vi "1000m_sub_frame.vi"(7 "Case select":string, 8 "felharmonikus N":i32=2, 9 "SNR window width [Hz]":dbl=0.4 format="%#_13g", 11 "path to binary file":path) -> (3 "output cluster":T1)   [LabVIEW 2017]
uses:
  <vilib>/Utility/file.llb/Read Delimited Spreadsheet (string).vi
  <vilib>/regexp/Match Regular Expression.xnode
panel:
  out "impulse szum/mean":cluster{"X":dbl, "Y":dbl}[](graph)
  out "Array":T2(array[cluster])
  out "header":T3
  out "impulse szum/time (bigger better)":cluster{"X":dbl, "Y":dbl}[](graph)
  out "X SNR 2":cluster{"X":dbl, "Y":dbl}[](graph)
  out "resultant SNR":cluster{"X":dbl, "Y":dbl}[](graph)
  out "X SNR":cluster{"X":dbl, "Y":dbl}[](graph)
  out "impulse mean":cluster{"X":dbl, "Y":dbl}[](graph)
  out "impulse sd":cluster{"X":dbl, "Y":dbl}[](graph)
  out "impulse szum":cluster{"X":dbl, "Y":dbl}[](graph)
  out "enable":bool
  out "end":timestamp
  out "start":timestamp
  out "state":string
  out "saved":string
  out "all rows":string[][](array[string])
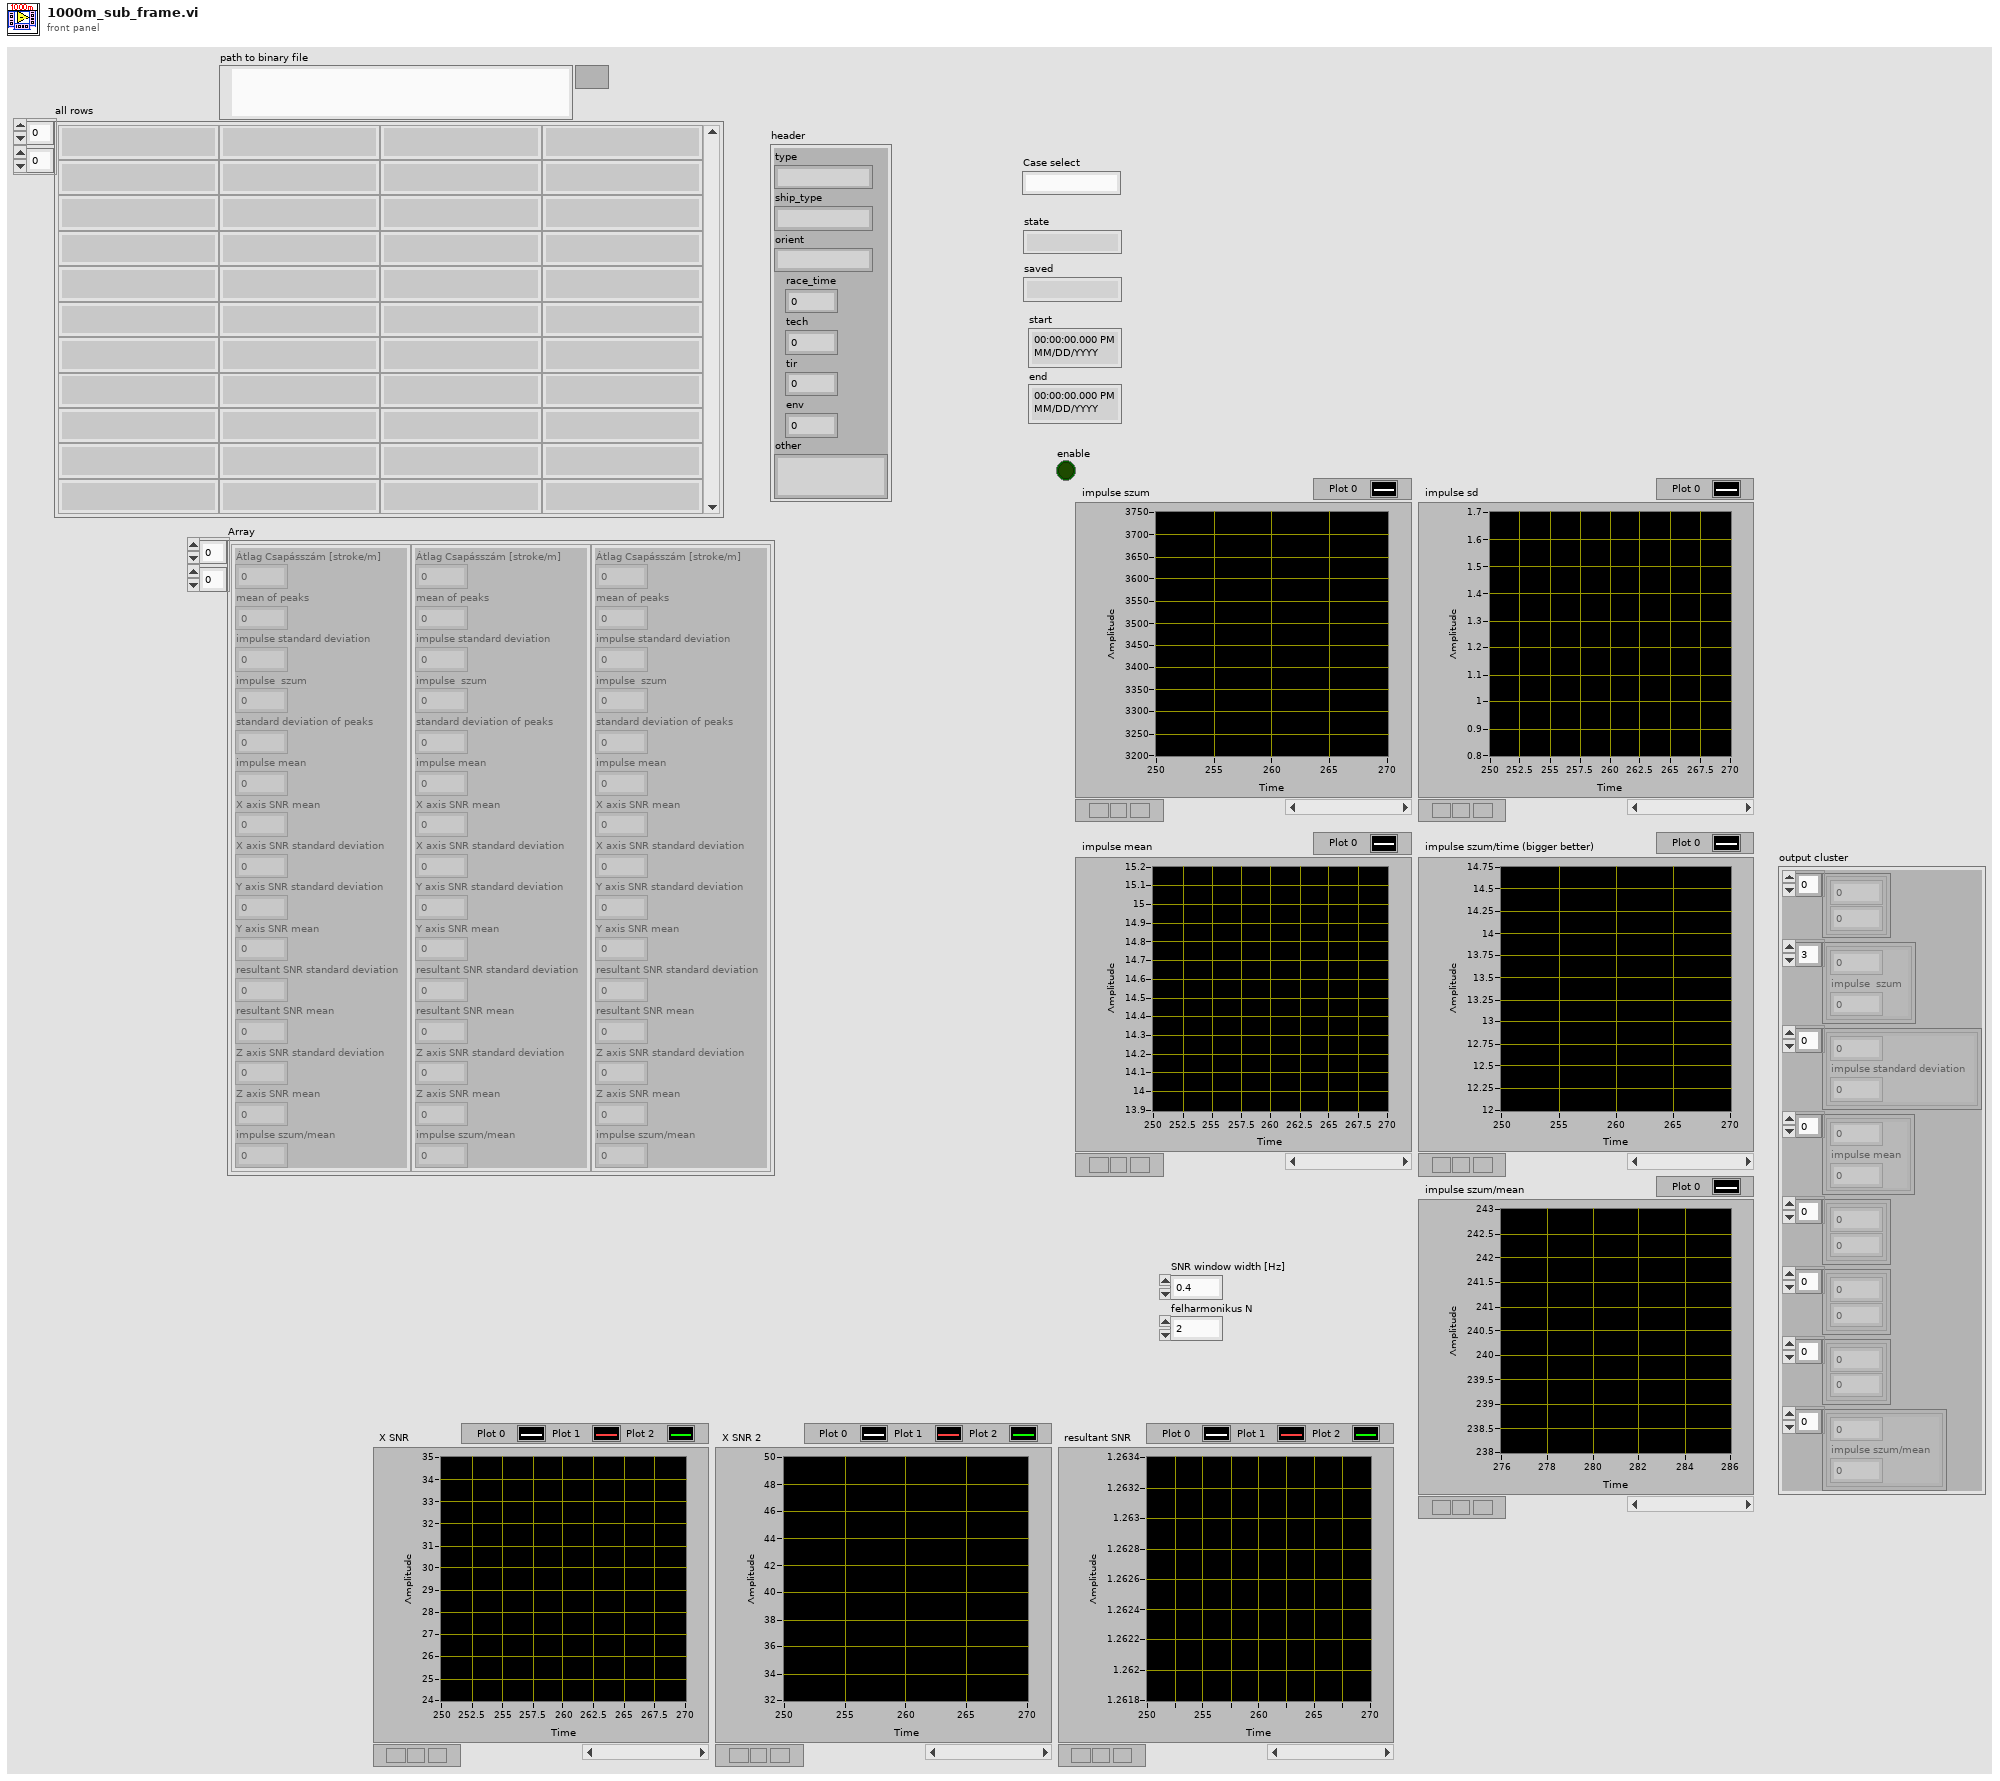
[diagram p1: front panel]
types:
  T1 = cluster{cluster{dbl, dbl}[], cluster{dbl, "impulse  szum":dbl}[], cluster{dbl, "impulse standard deviation":dbl}[], cluster{dbl, "impulse mean":dbl}[], cluster{dbl, dbl}[], cluster{dbl, dbl}[], cluster{dbl, dbl}[], cluster{dbl, "impulse szum/mean":dbl}[]}
  T2 = cluster{"Átlag Csapásszám [stroke/m]":dbl, "mean of peaks":dbl, "impulse standard deviation":dbl, "impulse  szum":dbl, "standard deviation of peaks":dbl, "impulse mean":dbl, "X axis SNR mean":dbl, "X axis SNR standard deviation":dbl, "Y axis SNR standard deviation":dbl, "Y axis SNR mean":dbl, "resultant SNR standard deviation":dbl, "resultant SNR mean":dbl, "Z axis SNR standard deviation":dbl, "Z axis SNR mean":dbl, "impulse szum/mean":dbl}[][]
  T3 = cluster{"type":string, "ship_type":string, "orient":string, "race_time":dbl, "tech":dbl, "tir":dbl, "env":dbl, "other":string}
  T4 = typedef "control_time_informations.ctl" = cluster{"starting time":timestamp, "ending time":timestamp, "dt[s]":dbl, "sampling rate [Hz]":dbl, "length":dbl}
  T5 = typedef "control_measurement_settings.ctl" = cluster{"sampling frequency [Hz]":dbl, "measurement interval [± g]":i32, "high precision?":bool, "number of pages":i32, "rate code":i32, "range code":i32, "id":i32}
  T6 = cluster{"statistics":cluster{"mean of x axis acceleration":dbl, "standard devation of x axis acceleration":dbl, "mean of y axis acceleration":dbl, "standard devation of y axis acceleration":dbl, "mean of z axis acceleration":dbl, "standard devation of z axis acceleration":dbl, "mean of magnitude of acceleration":dbl, "standard devation of magnitude of acceleration":dbl}, "time informations":T4, "actigraph settings":T5}
  T7 = cluster{"path to binary file":path, "Start Cursor":timestamp, "Sec":dbl, "crossing level":dbl, "threshold":dbl, "avg window size":i32, "peak detect width":i32, "invert":bool, "SNR window width [Hz]":dbl, "felharmonikus N":i32, "End cursor":timestamp}
  T8 = cluster{"Átlag Csapásszám [stroke/m]":dbl, "mean of peaks":dbl, "impulse standard deviation":dbl, "impulse  szum":dbl, "standard deviation of peaks":dbl, "impulse mean":dbl, "X axis SNR mean":dbl, "X axis SNR standard deviation":dbl, "Y axis SNR standard deviation":dbl, "Y axis SNR mean":dbl, "resultant SNR standard deviation":dbl, "resultant SNR mean":dbl, "Z axis SNR standard deviation":dbl, "Z axis SNR mean":dbl, "impulse szum/mean":dbl}
  T9 = cluster{"Átlag Csapásszám [stroke/m]":dbl, "mean of peaks":dbl, "impulse standard deviation":dbl, "impulse  szum":dbl, "standard deviation of peaks":dbl, "impulse mean":dbl, "X axis SNR mean":dbl, "X axis SNR standard deviation":dbl, "Y axis SNR standard deviation":dbl, "Y axis SNR mean":dbl, "resultant SNR standard deviation":dbl, "resultant SNR mean":dbl, "Z axis SNR standard deviation":dbl, "Z axis SNR mean":dbl, "impulse szum/mean":dbl}[]
  T10 = cluster{"Sec":dbl, "impulse standard deviation":dbl}
  T11 = cluster{cluster{"Sec":dbl, dbl}[], cluster{"Sec":dbl, "impulse  szum":dbl}[], cluster{"Sec":dbl, "impulse standard deviation":dbl}[], cluster{"Sec":dbl, "impulse mean":dbl}[], cluster{dbl, "SNR":dbl}[], cluster{dbl, "SNR":dbl}[], cluster{dbl, "SNR":dbl}[], cluster{"Sec":dbl, "impulse szum/mean":dbl}[]}
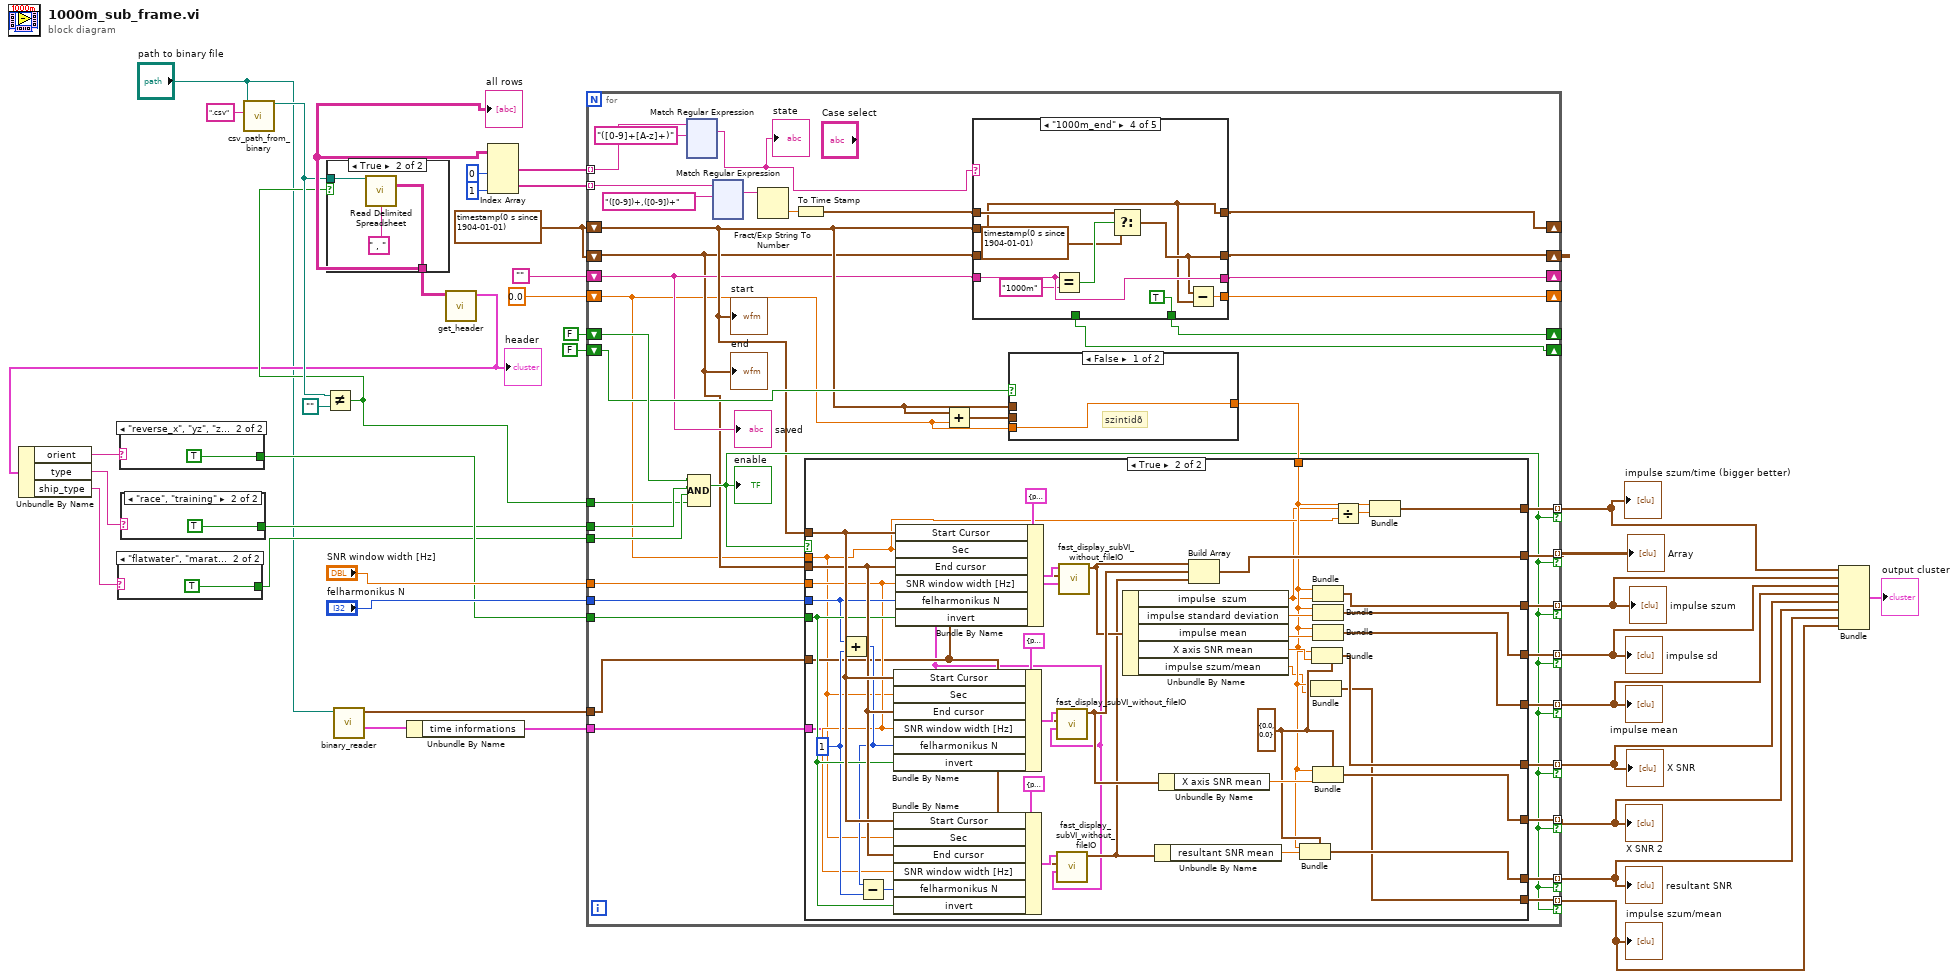
[diagram p0: block diagram]
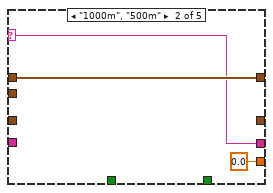
[diagram p3: hidden frame]
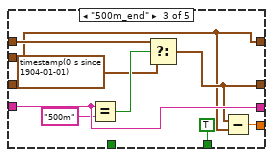
[diagram p4: hidden frame]
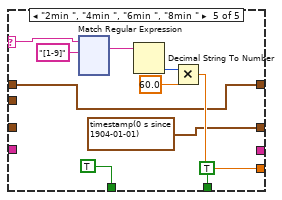
[diagram p5: hidden frame]
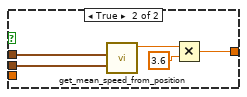
[diagram p6: hidden frame]
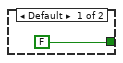
[diagram p9: hidden frame]
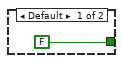
[diagram p10: hidden frame]
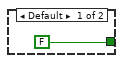
[diagram p11: hidden frame]
diagram:
  w10 = timestamp(0 s since 1904-01-01)
  n1 = call "csv_path_from_binary.vi"("extension"=".csv", "path to binary file"="path to binary file") -> ("path to spec. ext."=w14:path)  [unwired: 9 in]
  n2 = Not Equal?(x=w14, y=path "") -> (x != y?=w13:bool)
  n3 = case shown="True" w13 {
    tunnel: [_ w39] -> w15
    tunnel: w14 -> [_ w38]
    frame False {
    }
    frame True {
      n4 = call-poly <vilib>:"Read Delimited Spreadsheet.vi"("file path (dialog if empty)"=w38, "delimiter (\\t)"=" , " ("delimiter (\\t)")) -> ("all rows"=w39:string[][])  [unwired: 8 in, 5 out]
    }
  }
  "all rows" <- w15
  n5 = call "binary_reader.vi"("path to binary file"="path to binary file") -> ("Misc"=w3:T6, "3 axis acceleration in time"=w4:waveform(dbl)[])  [unwired: 6 in, 2 out]
  n6 = Unbundle By Name(w3) -> ("time informations"=w2:T4)
  n7 = call "get_header.vi"("all rows"=w15) -> ("header"=w11:T3)  [unwired: 10 in]
  "header" <- w11
  n8 = Unbundle By Name(w11) -> ("orient"=w29:string, "type"=w20:string, "ship_type"=w18:string)
  n9 = case shown="\"flatwater\", \"marathon\"" w18 {
    tunnel: [FALSE TRUE] -> w17
    frame Default {
    }
    frame "flatwater", "marathon" {
    }
  }
  n10 = case shown="\"reverse_x\", \"yz\", \"z\"" w29 {
    tunnel: [FALSE TRUE] -> w28
    frame Default {
    }
    frame "reverse_x", "yz", "z" {
    }
  }
  n11 = case shown="\"race\", \"training\"" w20 {
    tunnel: [FALSE TRUE] -> w19
    frame Default {
    }
    frame "race", "training" {
    }
  }
  n12 = Index Array(array=w15, index (col) #1=0 ("disabled index (col)"), index (col) #2=1 ("index (col)")) -> (element #1=w36:string[], element #2=w37:string[])  [unwired: 2 in]
  n13 = for {
    tunnel: w37 -> [w83] mode=indexing
    tunnel: w36 -> [w82] mode=indexing
    shift-right: [w51] -> _
    shift-left: w10 -> [w56]
    shift-right: [w52] -> _
    shift-left: w10 -> [w48]
    shift-right: [w50] -> _
    shift-left: "" -> [w55]
    shift-right: [w49] -> _
    shift-left: 0.0 ("Sec") -> [w47]
    shift-right: [w53] -> _
    shift-left: FALSE -> [w69]
    tunnel: "SNR window width [Hz]" -> [w80]
    tunnel: "felharmonikus N" -> [w79]
    tunnel: w28 -> [w78]
    tunnel: [w77] -> w8 mode=indexing if=w62
    tunnel: [w76] -> w26 mode=indexing if=w62
    tunnel: [w75] -> w25 mode=indexing if=w62
    tunnel: [w74] -> w24 mode=indexing if=w62
    tunnel: [w73] -> w23 mode=indexing if=w62
    tunnel: [w72] -> w22 mode=indexing if=w62
    tunnel: [w71] -> w21 mode=indexing if=w62
    tunnel: [w70] -> w27 mode=indexing if=w62
    tunnel: w19 -> [w68]
    tunnel: w17 -> [w67]
    tunnel: w13 -> [w66]
    shift-right: [w54] -> _
    shift-left: FALSE -> [w64]
    tunnel: [w63] -> w7 mode=indexing if=w62
    tunnel: w4 -> [w60]
    tunnel: w2 -> [w59]
    n14 = xnode "Match Regular Expression"("input string"=w82, "regular expression"="([0-9]+[A-z]+)") -> ("whole match"=w58:string)  [unwired: 4 in, 4 out]
    "state" <- w58
    n15 = Compound Arithmetic op=AND(w69, w68, w67, w66) -> (w62:bool)
    "enable" <- w62
    n16 = xnode "Match Regular Expression"("input string"=w83, "regular expression"="([0-9])+,([0-9])+") -> ("whole match"=w85:string)  [unwired: 4 in, 4 out]
    n17 = Fract/Exp String To Number(string=w85) -> (number=w84:dbl)  [unwired: 3 in, 1 out]
    n18 = To Time Stamp(1:w84) -> (0:w57:timestamp)
    n19 = Add(x=w56, y=w47) -> (x+y=w61:timestamp)
    n20 = case shown="\"1000m_end\"" w58 {
      selector: w58 -> [_ w91 _ _ w119]
      tunnel: [w87 w92 w93 w102 w114] -> w51
      tunnel: w57 -> [_ w92 w100 w109 w114]
      tunnel: [w88 _ w94 w103 timestamp(0 s since 1904-01-01) ("f")] -> w52
      tunnel: [w89 w91 w99 w108 _] -> w50
      tunnel: w55 -> [w89 _ w99 w108 _]
      tunnel: [_ 0.0 w95 w104 w115] -> w49
      tunnel: w48 -> [w88 _ _ _ _]
      tunnel: w56 -> [w87 _ w93 w102 _]
      tunnel: [_ _ TRUE TRUE TRUE] -> w53
      tunnel: [_ _ _ _ TRUE] -> w54
      frame Default {
      }
      frame "1000m", "500m" {
      }
      frame "500m_end" {
        n21 = Equal?(x=w99, y="500m") -> (x = y?=w101:bool)
        n22 = Select(t=w100, s=w101, f=timestamp(0 s since 1904-01-01)) -> (s? t:f=w94:timestamp)
        n23 = Subtract(x=w94, y=w93) -> (x-y=w95:dbl)
      }
      frame "1000m_end" {
        n24 = Equal?(x=w108, y="1000m") -> (x = y?=w110:bool)
        n25 = Select(t=w109, s=w110, f=timestamp(0 s since 1904-01-01)) -> (s? t:f=w103:timestamp)
        n26 = Subtract(x=w103, y=w102) -> (x-y=w104:dbl)
      }
      frame "2min ", "4min ", "6min ", "8min " {
        n27 = xnode "Match Regular Expression"("input string"=w119, "regular expression"="[1-9]") -> ("whole match"=w118:string)  [unwired: 4 in, 4 out]
        n28 = Decimal String To Number(string=w118) -> (number=w116:i32)  [unwired: 2 in, 1 out]
        n29 = Multiply(x=w116, y=60.0) -> (x*y=w115:dbl)
      }
    }
    n30 = case shown="False" w64 {
      tunnel: w56 -> [_ w237]
      tunnel: w61 -> [_ w236]
      tunnel: [w235 w239] -> w65
      tunnel: w47 -> [w235 _]
      frame False {
        # "szintidõ"
      }
      frame True {
        n31 = call "get_mean_speed_from_position.vi"("end"=w236, "start"=w237) -> ("mean speed [m/s]"=w240:dbl)  [unwired: 7 in, 2 out]
        n32 = Multiply(x=w240, y=3.6) -> (x*y=w239:dbl)
      }
    }
    n33 = case shown="True" w62 {
      tunnel: w56 -> [_ w273]
      tunnel: w48 -> [_ w272]
      tunnel: w47 -> [_ w243]
      tunnel: w80 -> [_ w266]
      tunnel: w79 -> [_ w270]
      tunnel: w78 -> [_ w271]
      tunnel: w65 -> [_ w248]
      tunnel: [_ w261] -> w77
      tunnel: [_ w260] -> w76
      tunnel: [_ w259] -> w75
      tunnel: [_ w258] -> w74
      tunnel: [_ w253] -> w73
      tunnel: [_ w252] -> w72
      tunnel: [_ w251] -> w71
      tunnel: [_ w249] -> w70
      tunnel: [_ w246] -> w63
      tunnel: w60 -> [_ w245]
      tunnel: w59 -> [_ w244]
      frame False {
      }
      frame True {
        w250 = cluster{dbl, "SNR":dbl} {0.0, "SNR"=0.0} ("cluster")
        w267 = 1
        n34 = Add(x=w270, y=w267) -> (x+y=w268:i32)
        n35 = Subtract(x=w268, y=w267) -> (x-y=w269:i32)
        n36 = Bundle By Name(cluster=T7 {"path to binary file"=path "C:/Users/Lenovo/Desktop/szakdoga/data", "Start Cursor"=timestamp(0 s since 1904-01-01), "Sec"=60.0, "crossing level"=0.0, "threshold"=0.35, "avg window size"=5, "peak detect width"=30, "invert"=FALSE, "SNR window width [Hz]"=0.5, "felharmonikus N"=2, "End cursor"=timestamp(0 s since 1904-01-01)} ("input cluster"), "Start Cursor"=w273, "Sec"=w243, "End cursor"=w272, "SNR window width [Hz]"=w266, "felharmonikus N"=w268, "invert"=w271) -> (w276:T7)
        n37 = Bundle By Name(cluster=T7 {"path to binary file"=path "C:/Users/Lenovo/Desktop/szakdoga/data", "Start Cursor"=timestamp(0 s since 1904-01-01), "Sec"=60.0, "crossing level"=0.0, "threshold"=0.35, "avg window size"=5, "peak detect width"=30, "invert"=FALSE, "SNR window width [Hz]"=0.5, "felharmonikus N"=2, "End cursor"=timestamp(0 s since 1904-01-01)} ("input cluster"), "Start Cursor"=w273, "Sec"=w243, "End cursor"=w272, "SNR window width [Hz]"=w266, "felharmonikus N"=w269, "invert"=w271) -> (w275:T7)
        n38 = Bundle By Name(cluster=T7 {"path to binary file"=path "C:/Users/Lenovo/Desktop/szakdoga/data", "Start Cursor"=timestamp(0 s since 1904-01-01), "Sec"=60.0, "crossing level"=0.0, "threshold"=0.35, "avg window size"=5, "peak detect width"=30, "invert"=FALSE, "SNR window width [Hz]"=0.5, "felharmonikus N"=2, "End cursor"=timestamp(0 s since 1904-01-01)} ("input cluster"), "Start Cursor"=w273, "Sec"=w243, "End cursor"=w272, "SNR window width [Hz]"=w266, "felharmonikus N"=w270, "invert"=w271) -> (w279:T7)
        n39 = call "fast_display_subVI_without_fileIO.vi"("time informations"=w244, "acc waveform array"=w245, "input cluster"=w276) -> ("data cluster"=w263:T8)  [unwired: 8 in]
        n40 = call "fast_display_subVI_without_fileIO.vi"("time informations"=w244, "acc waveform array"=w245, "input cluster"=w275) -> ("data cluster"=w254:T8)  [unwired: 8 in]
        n41 = call "fast_display_subVI_without_fileIO.vi"("time informations"=w244, "acc waveform array"=w245, "input cluster"=w279) -> ("data cluster"=w262:T8)  [unwired: 8 in]
        n42 = Unbundle By Name(w262) -> ("impulse  szum"=w242:dbl, "impulse standard deviation"=w264:dbl, "impulse mean"=w265:dbl, "X axis SNR mean"=w257:dbl, "impulse szum/mean"=w247:dbl)
        n43 = Unbundle By Name(w254) -> ("resultant SNR mean"=w255:dbl)
        n44 = Unbundle By Name(w263) -> ("X axis SNR mean"=w256:dbl)
        n45 = Build Array(w262, w263, w254) -> (w261:T9)
        n46 = Bundle(cluster=w250, w248, "SNR"=w255) -> (w251:cluster{dbl, "SNR":dbl})
        n47 = Bundle("Sec"=w248, "impulse szum/mean"=w247) -> (w246:cluster{"Sec":dbl, "impulse szum/mean":dbl})  [unwired: 1 in]
        n48 = Bundle(cluster=w250, w248, "SNR"=w257) -> (w253:cluster{dbl, "SNR":dbl})
        n49 = Bundle("Sec"=w248, "impulse  szum"=w242) -> (w260:cluster{"Sec":dbl, "impulse  szum":dbl})  [unwired: 1 in]
        n50 = Bundle("Sec"=w248, "impulse standard deviation"=w264) -> (w259:T10)  [unwired: 1 in]
        n51 = Bundle("Sec"=w248, "impulse mean"=w265) -> (w258:cluster{"Sec":dbl, "impulse mean":dbl})  [unwired: 1 in]
        n52 = Bundle(cluster=w250, w248, "SNR"=w256) -> (w252:cluster{dbl, "SNR":dbl})
        n53 = Divide(x=w242, y=w243) -> (x/y=w241:dbl)
        n54 = Bundle("Sec"=w248, w241) -> (w249:cluster{"Sec":dbl, dbl})  [unwired: 1 in]
      }
    }
    "saved" <- w55
    "start" <- w56
    "end" <- w48
  }
  "impulse szum" <- w26
  "impulse sd" <- w25
  "impulse mean" <- w24
  "X SNR" <- w23
  "resultant SNR" <- w21
  "X SNR 2" <- w22
  "impulse szum/time (bigger better)" <- w27
  "Array" <- w8
  "impulse szum/mean" <- w7
  n55 = Bundle(w27, w26, w25, w24, w23, w22, w21, w7) -> (→"output cluster":T11)  [unwired: 1 in]
